vi "CR FitEllipse.vi"(8 "Image Name":string="ellipse2", 9 "r":dbl=100.0, 10 "rough center":cluster{"Pos. X":i32, "Pos. Y":i32}, 11 "Image Src":T1) -> (2 "Valid Fit":bool, 3 "Ellipse 2":T2 {"Minor Axis"."Point 2"."Y" format="%.2f"; "Minor Axis"."Point 2"."X" format="%.2f"; "Minor Axis"."Point 1"."Y" format="%.2f"; "Minor Axis"."Point 1"."X" format="%.2f"; "Major Axis"."Point 2"."Y" format="%.2f"; "Major Axis"."Point 2"."X" format="%.2f"; "Major Axis"."Point 1"."Y" format="%.2f"; "Major Axis"."Point 1"."X" format="%.2f"; "Center"."Y" format="%.2f"; "Center"."X" format="%.2f"})   [LabVIEW 2011]
uses:
  <vilib>/vision/Image Controls.llb/IMAQ Image.ctl
  <vilib>/vision/NI_Vision_Development_Module.lvlib
panel:
  out "Image Out":T1
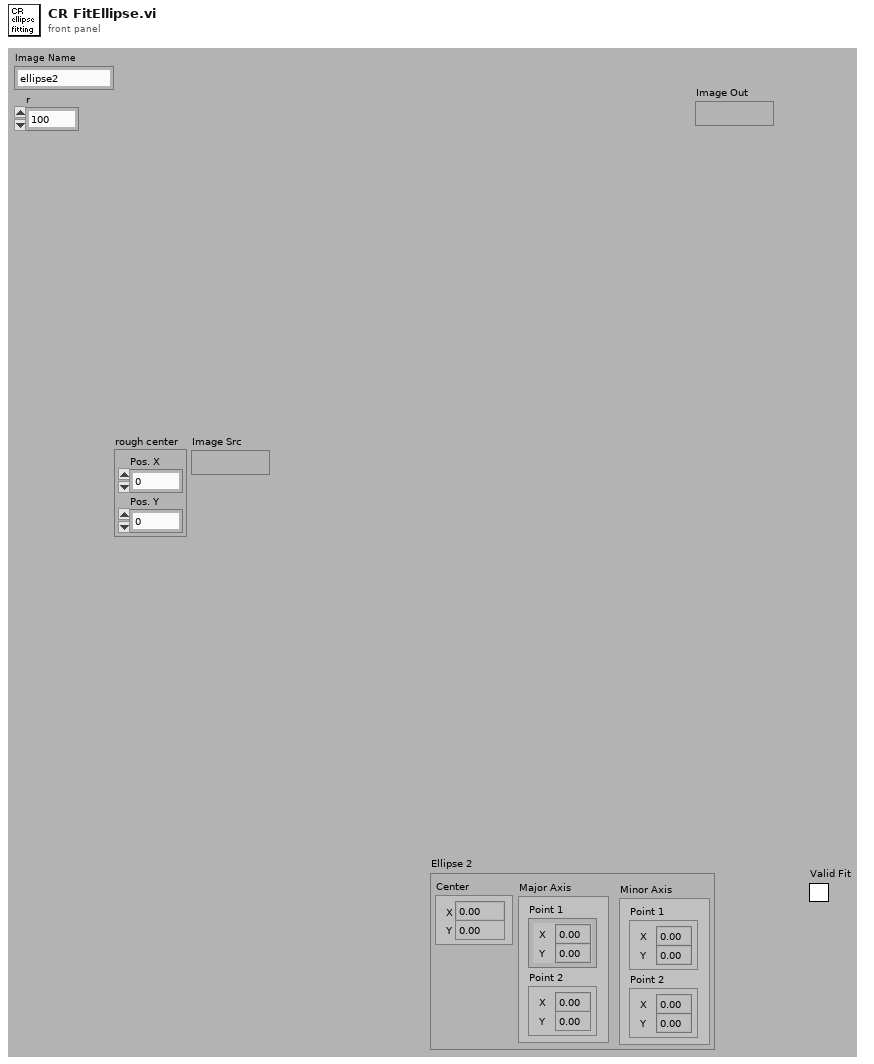
[diagram p1: front panel]
types:
  T1 = typedef "IMAQ Image.ctl" = refnum<image>
  T2 = cluster{"Center":cluster{"X":sgl, "Y":sgl}, "Major Axis":cluster{"Point 1":cluster{"X":sgl, "Y":sgl}, "Point 2":cluster{"X":sgl, "Y":sgl}}, "Minor Axis":cluster{"Point 1":cluster{"X":sgl, "Y":sgl}, "Point 2":cluster{"X":sgl, "Y":sgl}}}
  T3 = enum32{"Differentiation", "Gradient", "Prewitt", "Roberts", "Sigma", "Sobel"}
  T4 = typedef "Image Type" = u32
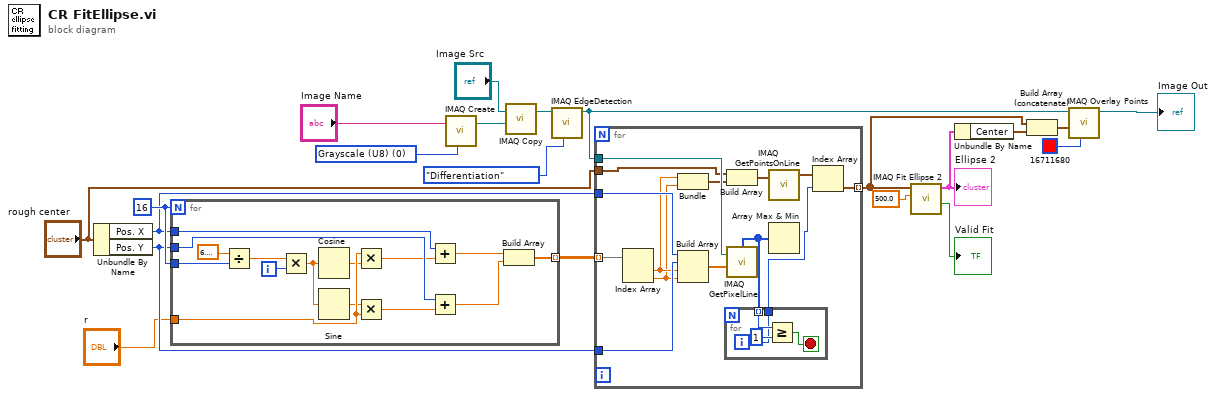
[diagram p0: block diagram]
diagram:
  w5 = 16
  w21 = T4 0 items=["Grayscale (U8)", "Grayscale (I16)", "Grayscale (SGL)", "Complex (CSG)", "RGB (U32)", "HSL (U32)", "RGB (U64)", "Grayscale (U16)"] ("Image Type")
  n1 = Unbundle By Name("rough center") -> ("Pos. X"=w4:i32, "Pos. Y"=w3:i32)
  n2 = for {
    N: w5 -> [_]
    tunnel: w5 -> [w36]
    tunnel: [w32] -> w1 mode=indexing
    tunnel: w4 -> [w31]
    tunnel: w3 -> [w29]
    tunnel: "r" -> [w26]
    i -> [w27]
    n3 = Divide(x=6.283185307179586, y=w36) -> (x/y=w34:dbl)
    n4 = Multiply(x=w34, y=w27) -> (x*y=w33:dbl)
    n5 = Cosine(x=w33) -> (cos(x)=w23:dbl)
    n6 = Sine(x=w33) -> (sin(x)=w25:dbl)
    n7 = Multiply(x=w26, y=w23) -> (x*y=w22:dbl)
    n8 = Multiply(x=w25, y=w26) -> (x*y=w24:dbl)
    n9 = Add(x=w31, y=w22) -> (x+y=w30:dbl)
    n10 = Add(x=w29, y=w24) -> (x+y=w28:dbl)
    n11 = Build Array(w30, w28) -> (w32:dbl[])
  }
  n12 = call "IMAQ Create"("Image Name"="Image Name", "Image Type"=w21) -> ("New Image"=w19:T1)  [unwired: 2 in, 2 out]
  n13 = call "IMAQ Copy"("Image Dst"=w19, "Image Src"="Image Src") -> ("Image Dst Out"=w18:T1)  [unwired: 1 in, 4 out]
  n14 = call "IMAQ EdgeDetection"("Method"=T3."Differentiation", "Image Src"=w18) -> ("Image Dst Out"=w10:T1)  [unwired: 4 in, 5 out]
  n15 = for {
    tunnel: w1 -> [w50] mode=indexing
    tunnel: w4 -> [w49]
    tunnel: w3 -> [w48]
    tunnel: w10 -> [w47]
    tunnel: "rough center" -> [w42]
    tunnel: [w39] -> w6 mode=indexing
    n16 = Index Array(array=w50) -> (element #1=w45:dbl, element #2=w44:dbl)  [unwired: 2 in]
    n17 = Bundle(w45, w44) -> (w43:cluster{dbl, dbl})  [unwired: 1 out]
    n18 = Build Array(w49, w48, w45, w44) -> (w46:dbl[])
    n19 = Build Array(w42, w43) -> (w41:cluster{"Pos. X":dbl, "Pos. Y":dbl}[])
    n20 = call "IMAQ GetPixelLine"("Line Coordinates"=w46, "Image"=w47) -> ("Pixels Line (U8)"=w38:u8[])  [unwired: 1 in, 5 out]
    n21 = for {
      tunnel: w38 -> [w54] mode=indexing
      tunnel: [w51] -> w37
      i -> [w51]
      stop <- w52 stop-if-true
      n22 = Greater Or Equal?(x=w54, y=u8 1) -> (x >= y?=w52:bool)
    }
    n23 = call "IMAQ GetPointsOnLine"("Endpoints"=w41) -> ("Points of the Line"=w40:cluster{"X":i32, "Y":i32}[])  [unwired: 1 in, 2 out]
    n24 = Array Max & Min(array=w38) -> ()  [unwired: 4 out]
    n25 = Index Array(array=w40, index=w37) -> (element=w39:cluster{"X":i32, "Y":i32})
  }
  n26 = call "IMAQ Fit Ellipse 2"("Minimum Score"=500.0, "Radial Points"=w6) -> ("Valid Fit"=→"Valid Fit":bool, "Ellipse"=w13:T2)  [unwired: 4 in, 4 out]
  "Ellipse 2" <- w13
  n27 = Unbundle By Name(w13) -> ("Center"=w12:cluster{"X":sgl, "Y":sgl})
  n28 = Build Array (concatenate)(w6, w12) -> (w11:cluster{"X":sgl, "Y":sgl}[])
  n29 = call "IMAQ Overlay Points"("Color"=u32 16711680, "Array of Points"=w11, "Image"=w10) -> ("Image Out"=→"Image Out":T1)  [unwired: 3 in, 5 out]
